vi "sum.vi"(7 "numeric array":fxp<+/-,32,32>[](array[numeric])=[0.0, 0.0, 0.0, 0.0, 0.0, 0.0, 0.0, 0.0, 0.0, 0.0, 0.0, 0.0, 0.0, 0.0, 0.0, 0.0, 0.0, 0.0, 0.0, 0.0, 0.0, 0.0, 0.0, 0.0, 0.0, 0.0, 0.0, 0.0, 0.0, 0.0, 0.0, 0.0]) -> (1 "temp":i32, 3 "Numeric":i32)   [LabVIEW 2021]
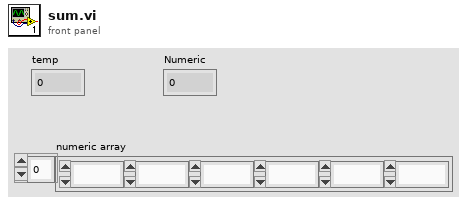
[diagram p1: front panel]
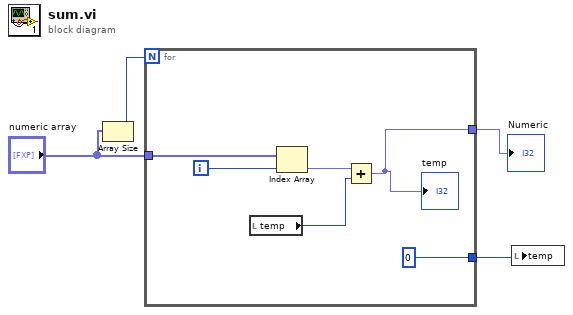
[diagram p0: block diagram]
diagram:
  n1 = Array Size(array="numeric array") -> (size(s)=w4:i32)
  n2 = for {
    N: w4 -> [_]
    tunnel: "numeric array" -> [w10]
    tunnel: [w7] -> w2
    tunnel: [0] -> w1
    i -> [w6]
    n3 = local read "temp"() -> (w8:i32)
    n4 = Index Array(array=w10, index=w6) -> (element=w9:fxp<+/-,32,32>)
    n5 = Add(x=w9, y=w8) -> (x+y=w7:fxp<+/-,33,33>)
    "temp" <- w7
  }
  "Numeric" <- w2
  n6 = local write "temp"(w1) -> ()
